vi "calc_phase_map_joe.vi"(4 "u8_ar_image_pixel_array":u8[][][](array[numeric]), 5 "image name":string="fringe") -> (0 "raw phase map array":u8[][](array[numeric]), 1 "phase map":T1(plugin-control))   [LabVIEW 2011]
uses:
  global_vars.vi
  <vilib>/express/express arith-compare/Formula/XNode/ExpressFormulaBlockNode.xnode
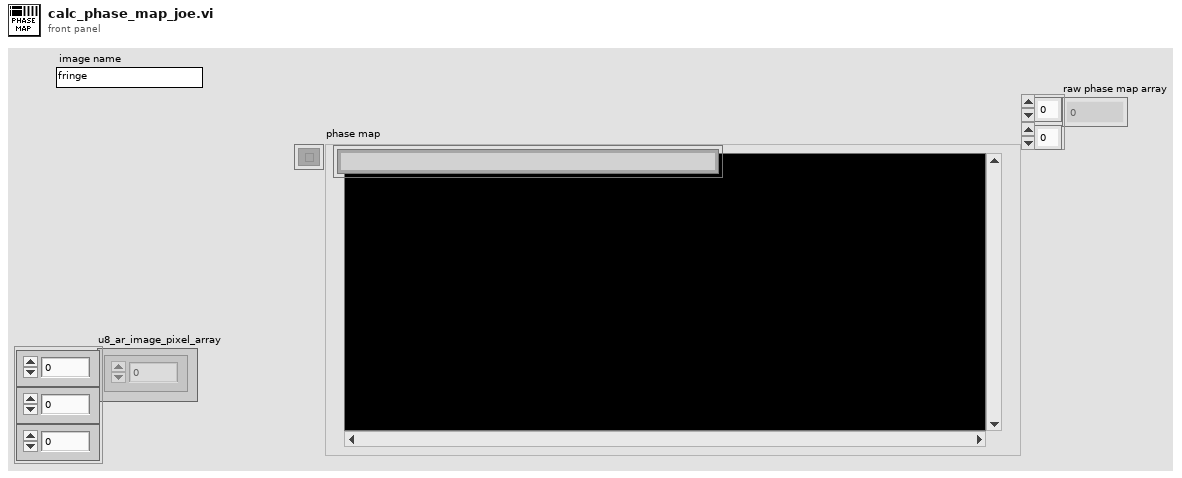
[diagram p1: front panel]
types:
  T1 = typedef "IMAQ Image.ctl" = refnum<image>
  T2 = typedef "Image Type" = u32
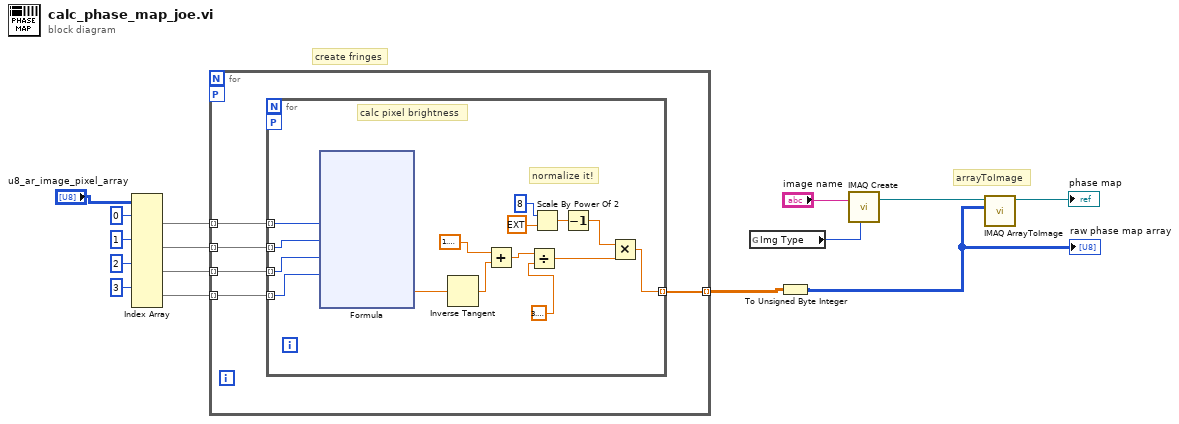
[diagram p0: block diagram]
diagram:
  # "create fringes"
  # "arrayToImage"
  n1 = Index Array(array="u8_ar_image_pixel_array", index (dim 0) #1=0 ("index (page)"), index (dim 0) #2=1 ("index (page)"), index (dim 0) #3=2 ("index (page)"), index (dim 0) #4=3 ("index (page)")) -> (element #1=w9:u8[][], element #2=w8:u8[][], element #3=w7:u8[][], element #4=w6:u8[][])  [unwired: 8 in]
  n2 = for {
    tunnel: w9 -> [w20] mode=indexing
    tunnel: w8 -> [w19] mode=indexing
    tunnel: w7 -> [w18] mode=indexing
    tunnel: w6 -> [w17] mode=indexing
    tunnel: [w16] -> w5 mode=indexing
    workers-P: _ -> [_]
    n3 = for {
      tunnel: w20 -> [w35] mode=indexing
      tunnel: w19 -> [w34] mode=indexing
      tunnel: w18 -> [w33] mode=indexing
      tunnel: w17 -> [w32] mode=indexing
      tunnel: [w22] -> w16 mode=indexing
      workers-P: _ -> [_]
      # "normalize it!"
      # "calc pixel brightness"
      n4 = xnode ("Formula")("A1"=w35, "A2"=w34, "A3"=w33, "A4"=w32) -> ("Result"=w31:dbl)  [unwired: 1 in, 1 out]
      n5 = Inverse Tangent(1:w31) -> (0:w28:dbl)
      n6 = Add(x=1.5707963267948966, y=w28) -> (x+y=w26:dbl)
      n7 = Divide(x=w26, y=3.141592653589793) -> (x/y=w23:dbl)
      n8 = Scale By Power Of 2(n=8, x=ext 1.0) -> (x*2^n=w29:ext)
      n9 = Decrement(x=w29) -> (x-1=w24:ext)
      n10 = Multiply(x=w24, y=w23) -> (x*y=w22:ext)
    }
  }
  n11 = global read "global_vars.vi" "Img Type"() -> (w1:T2)
  n12 = To Unsigned Byte Integer(number=w5) -> (unsigned 8bit integer=w3:u8[][])
  "raw phase map array" <- w3
  n13 = call "IMAQ Create"("Image Name"="image name", "Image Type"=w1) -> ("New Image"=w2:T1)  [unwired: 2 in, 2 out]
  n14 = call "IMAQ ArrayToImage"("Image Pixels (U8)"=w3, "Image"=w2) -> ("Image Out"=→"phase map":T1)  [unwired: 8 in, 1 out]
